vi "Update Parameters.vi"(8 "error in (no error)":errorcluster, 10 "Parameters":refnum<class "Parameter.lvclass">[](array[class]), 11 "WriteCommand in":refnum<class "WriteCommand.lvclass">) -> (0 "error out":errorcluster, 3 "WriteCommand out":refnum<class "WriteCommand.lvclass">)   [LabVIEW 2023, in "HAF.lvlib" / "WriteCommand.lvclass"]
doc: "Adds to, or updates in, the existing collection of Parameters on the Command. Returns the number added and updated."
uses:
  WriteCommand.lvclass
  Parameter/Parameter.lvclass
  WriteCommand.lvclass/WriteCommand.ctl
panel:
  out "Updated Count":u32
  out "Added Count":u32
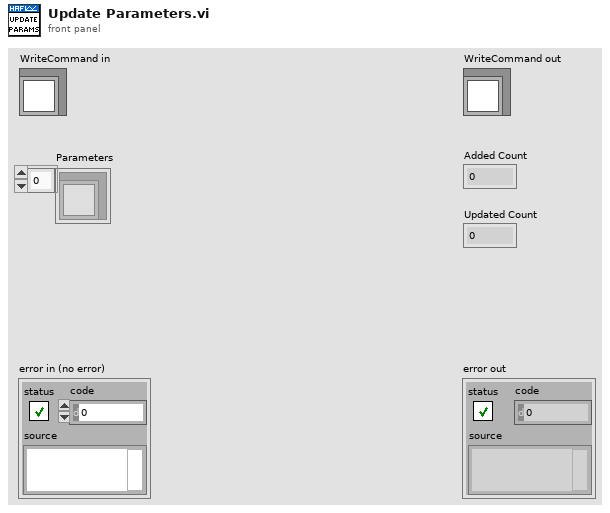
[diagram p1: front panel]
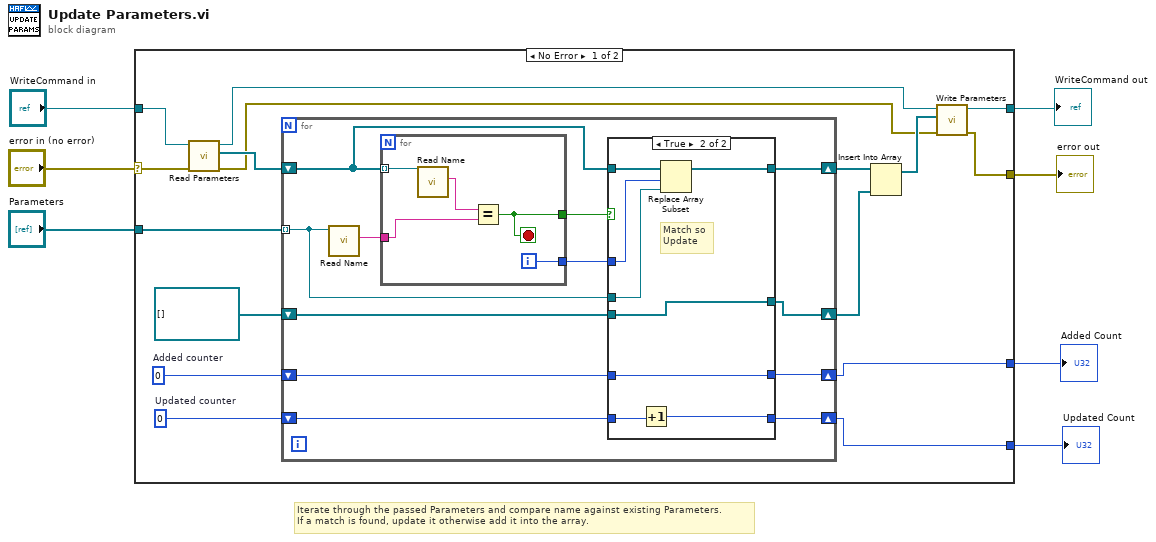
[diagram p0: block diagram]
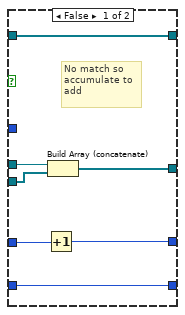
[diagram p2: hidden frame]
diagram:
  # "Iterate through the passed Parameters and compare name against existing Parameters.\nIf a match is found, update it otherwise add it into the array."
  n1 = case shown="No Error" "error in (no error)" {
    selector: "error in (no error)" -> [w22 w57]
    tunnel: [w10 w57] -> w3
    tunnel: [w11 w56] -> w4
    tunnel: "WriteCommand in" -> [w23 w56]
    tunnel: "Parameters" -> [w20 _]
    tunnel: [w9 _] -> w2
    tunnel: [w8 _] -> w1
    frame No Error {
      w17 = u32 0  # Updated counter
      w18 = u32 0  # Added counter
      n2 = call-dynamic "Read Parameters.vi"("error in (no error)"=w22, "WriteCommand in"=w23) -> ("error out"=w13:errorcluster, "Parameters"=w21:refnum<class "Parameter.lvclass">[], "WriteCommand out"=w12:refnum<class "WriteCommand.lvclass">)  [unwired: 7 in]
      n3 = for {
        shift-right: [w27] -> w16
        shift-left: w21 -> [w34]
        tunnel: w20 -> [w31] mode=indexing
        shift-right: [w26] -> w15
        shift-left: refnum<class "Parameter.lvclass">[] [] -> [w30]
        shift-right: [w25] -> w9
        shift-left: w18 -> [w29]
        shift-right: [w24] -> w8
        shift-left: w17 -> [w28]
        n4 = call-dynamic "Read Name.vi"("Parameter in"=w31) -> ("Name"=w35:string)  [unwired: 8 in, 2 out]
        n5 = for {
          tunnel: w35 -> [w53]
          tunnel: w34 -> [w55] mode=indexing
          tunnel: [w52] -> w33
          tunnel: [w51] -> w32
          i -> [w51]
          stop <- w52 stop-if-true
          n6 = call-dynamic "Read Name.vi"("Parameter in"=w55) -> ("Name"=w54:string)  [unwired: 8 in, 2 out]
          n7 = Equal?(x=w54, y=w53) -> (x = y?=w52:bool)
        }
        n8 = case shown="True" w33 {
          tunnel: w34 -> [w42 w50]
          tunnel: w32 -> [_ w49]
          tunnel: w31 -> [w41 w48]
          tunnel: w30 -> [w40 w46]
          tunnel: w29 -> [w38 w45]
          tunnel: w28 -> [w36 w44]
          tunnel: [w42 w47] -> w27
          tunnel: [w39 w46] -> w26
          tunnel: [w37 w45] -> w25
          tunnel: [w36 w43] -> w24
          frame False {
            # "No match so\naccumulate to\nadd"
            n9 = Increment(x=w38) -> (x+1=w37:u32)
            n10 = Build Array (concatenate)(w41, w40) -> (w39:refnum<class "Parameter.lvclass">[])
          }
          frame True {
            # "Match so\nUpdate"
            n11 = Increment(x=w44) -> (x+1=w43:u32)
            n12 = Replace Array Subset(array=w50, new element=w48, index=w49) -> (w47:refnum<class "Parameter.lvclass">[])
          }
        }
      }
      n13 = Insert Into Array(array=w16, new element=w15) -> (w14:refnum<class "Parameter.lvclass">[])  [unwired: 1 in]
      n14 = call-dynamic "Write Parameters.vi"("error in (no error)"=w13, "Parameters"=w14, "WriteCommand in"=w12) -> ("error out"=w10:errorcluster, "WriteCommand out"=w11:refnum<class "WriteCommand.lvclass">)  [unwired: 7 in]
    }
    frame Error {
    }
  }
  "error out" <- w3
  "WriteCommand out" <- w4
  "Added Count" <- w2
  "Updated Count" <- w1
